vi "test_riccat_01Ni.vi"() -> (3 "All Tests Passed":bool)   [LabVIEW 2019]
uses:
  <vilib>/Analysis/Matrix/Datatypes/RealMatrix.ctl
  <vilib>/Rock Robotics/WPI/ThirdParty/JAS_Junk/TrajLib/Trajectory_Library.lvlib
  <vilib>/Analysis/Matrix/NI_Matrix.lvlib
panel:
  out "N1":T1
  out "R1":T1
  out "Q1":T1
  in  "AREF":T1=[[0.25, 1.0, 0.0, 0.0], [0.0, 0.0, 1.0, 0.0], [0.0, 0.0, 0.0, 1.0], [0.0, 0.0, 0.0, 0.0]]
  out "error out 2":errorcluster
  out "Pos Semi Definite":bool
  out "C":T1
  out "Q_Chk_Passed":bool
  out "Q Check":T1
  out "Stable Bad":bool
  out "Bad":bool
  out "Eigenvalues":cdb[](array[numeric])
  out "error out":errorcluster
  out "Error":bool
  out "Iterations":i32
  out "Elapsed \nTime MS":dbl
  out "ZERO":T1
  out "X  Answer":T1
  in  "R":T1=[[0.25]]
  in  "Q":T1=[[1.0, 0.0, 0.0, 0.0], [0.0, 0.0, 0.0, 0.0], [0.0, 0.0, 0.0, 0.0], [0.0, 0.0, 0.0, 0.0]]
  in  "B":T1=[[0.0], [0.0], [0.0], [1.0]]
  in  "A":T1=[[0.5, 1.0, 0.0, 0.0], [0.0, 0.0, 1.0, 0.0], [0.0, 0.0, 0.0, 1.0], [0.0, 0.0, 0.0, 0.0]]
  # "Test 1: non-invertible A\n  // Example 2 of \"On the Numerical Solution of the Discrete-Time Algebraic\n  // Riccati Equation\""
  # "int n1 = 4, m1 = 1;"
  # "Example = F"
  # "MatrixXd A1(n1, n1), B1(n1, m1), Q1(n1, n1), R1(m1, m1);"
  # "A1 << 0.5, 1, 0, 0, \n          0, 0, 1, 0, \n          0, 0, 0, 1, \n          0, 0, 0, 0;"
  # "B1 << 0, \n        0, \n        0, \n        1;"
  # "Example G1"
  # "Example H"
  # "Solution weight ??"
  # "Q1 << 1, 0, 0, 0, \n        0, 0, 0, 0, \n        0, 0, 0, 0, \n        0, 0, 0, 0;"
  # "Example G2"
  # "Cost ??"
  # "R1 << 0.25;"
  # "0.25, 1, 0, 0, \n0,      0, 1, 0, \n0,      0, 0, 1, \n0,      0, 0, 0;"
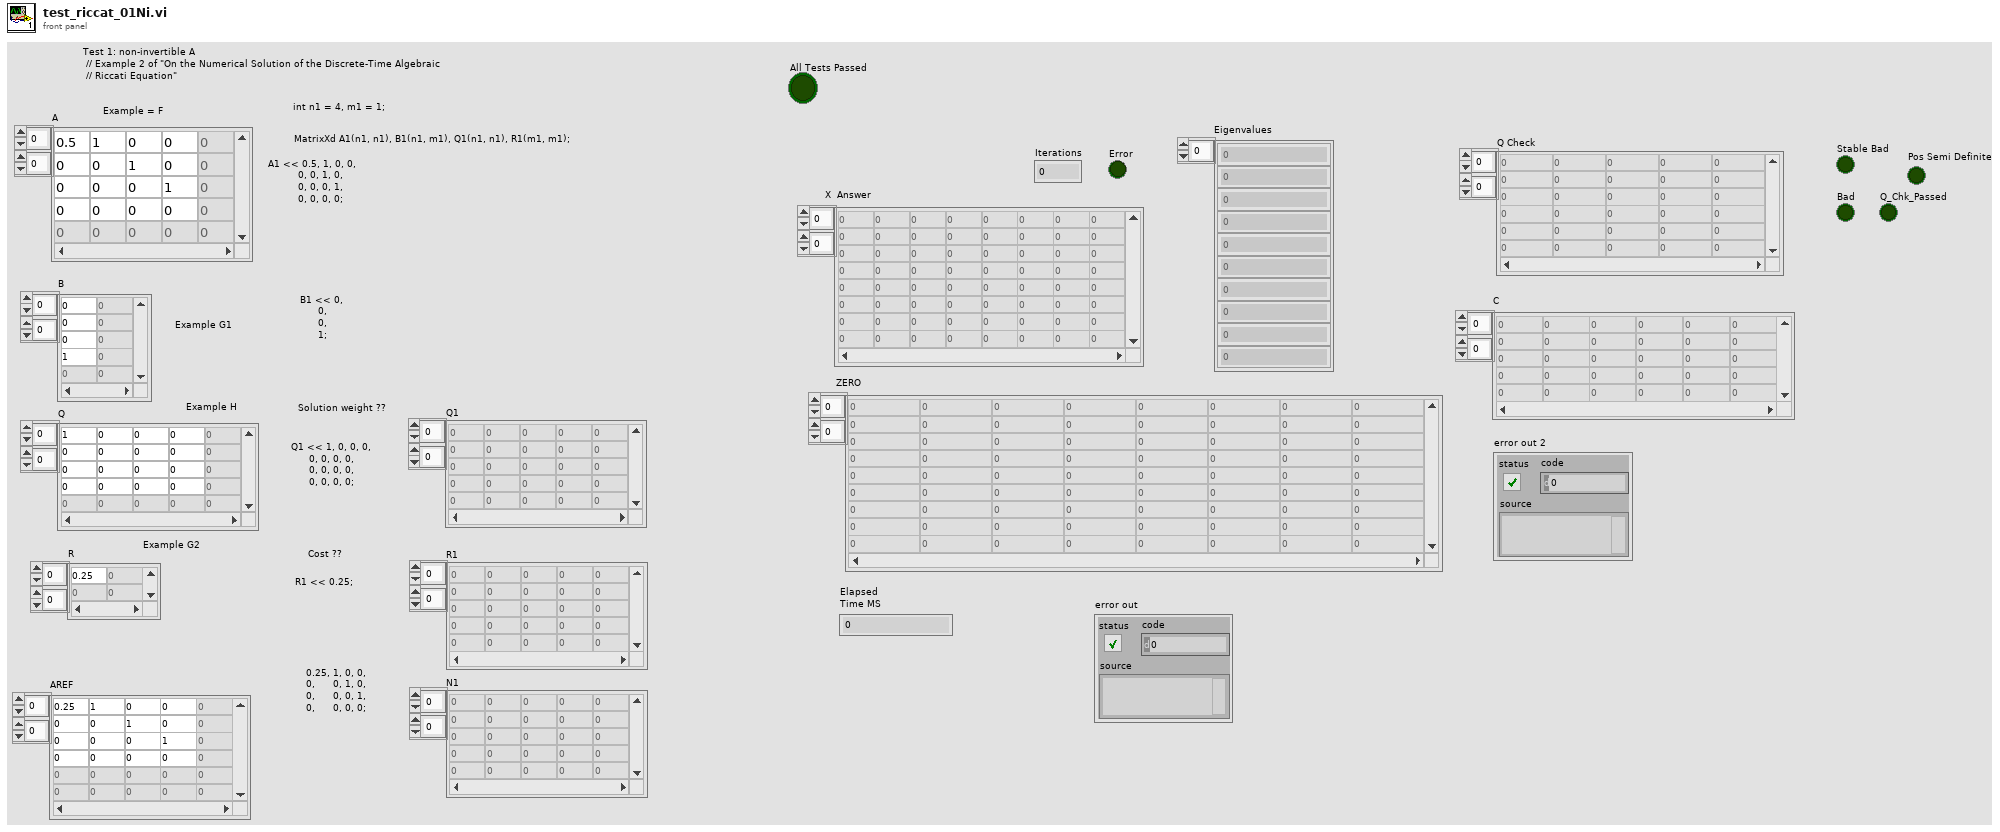
[diagram p1: front panel]
types:
  T1 = typedef "NI_Matrix.lvlib/RealMatrix.ctl" = dbl[][]
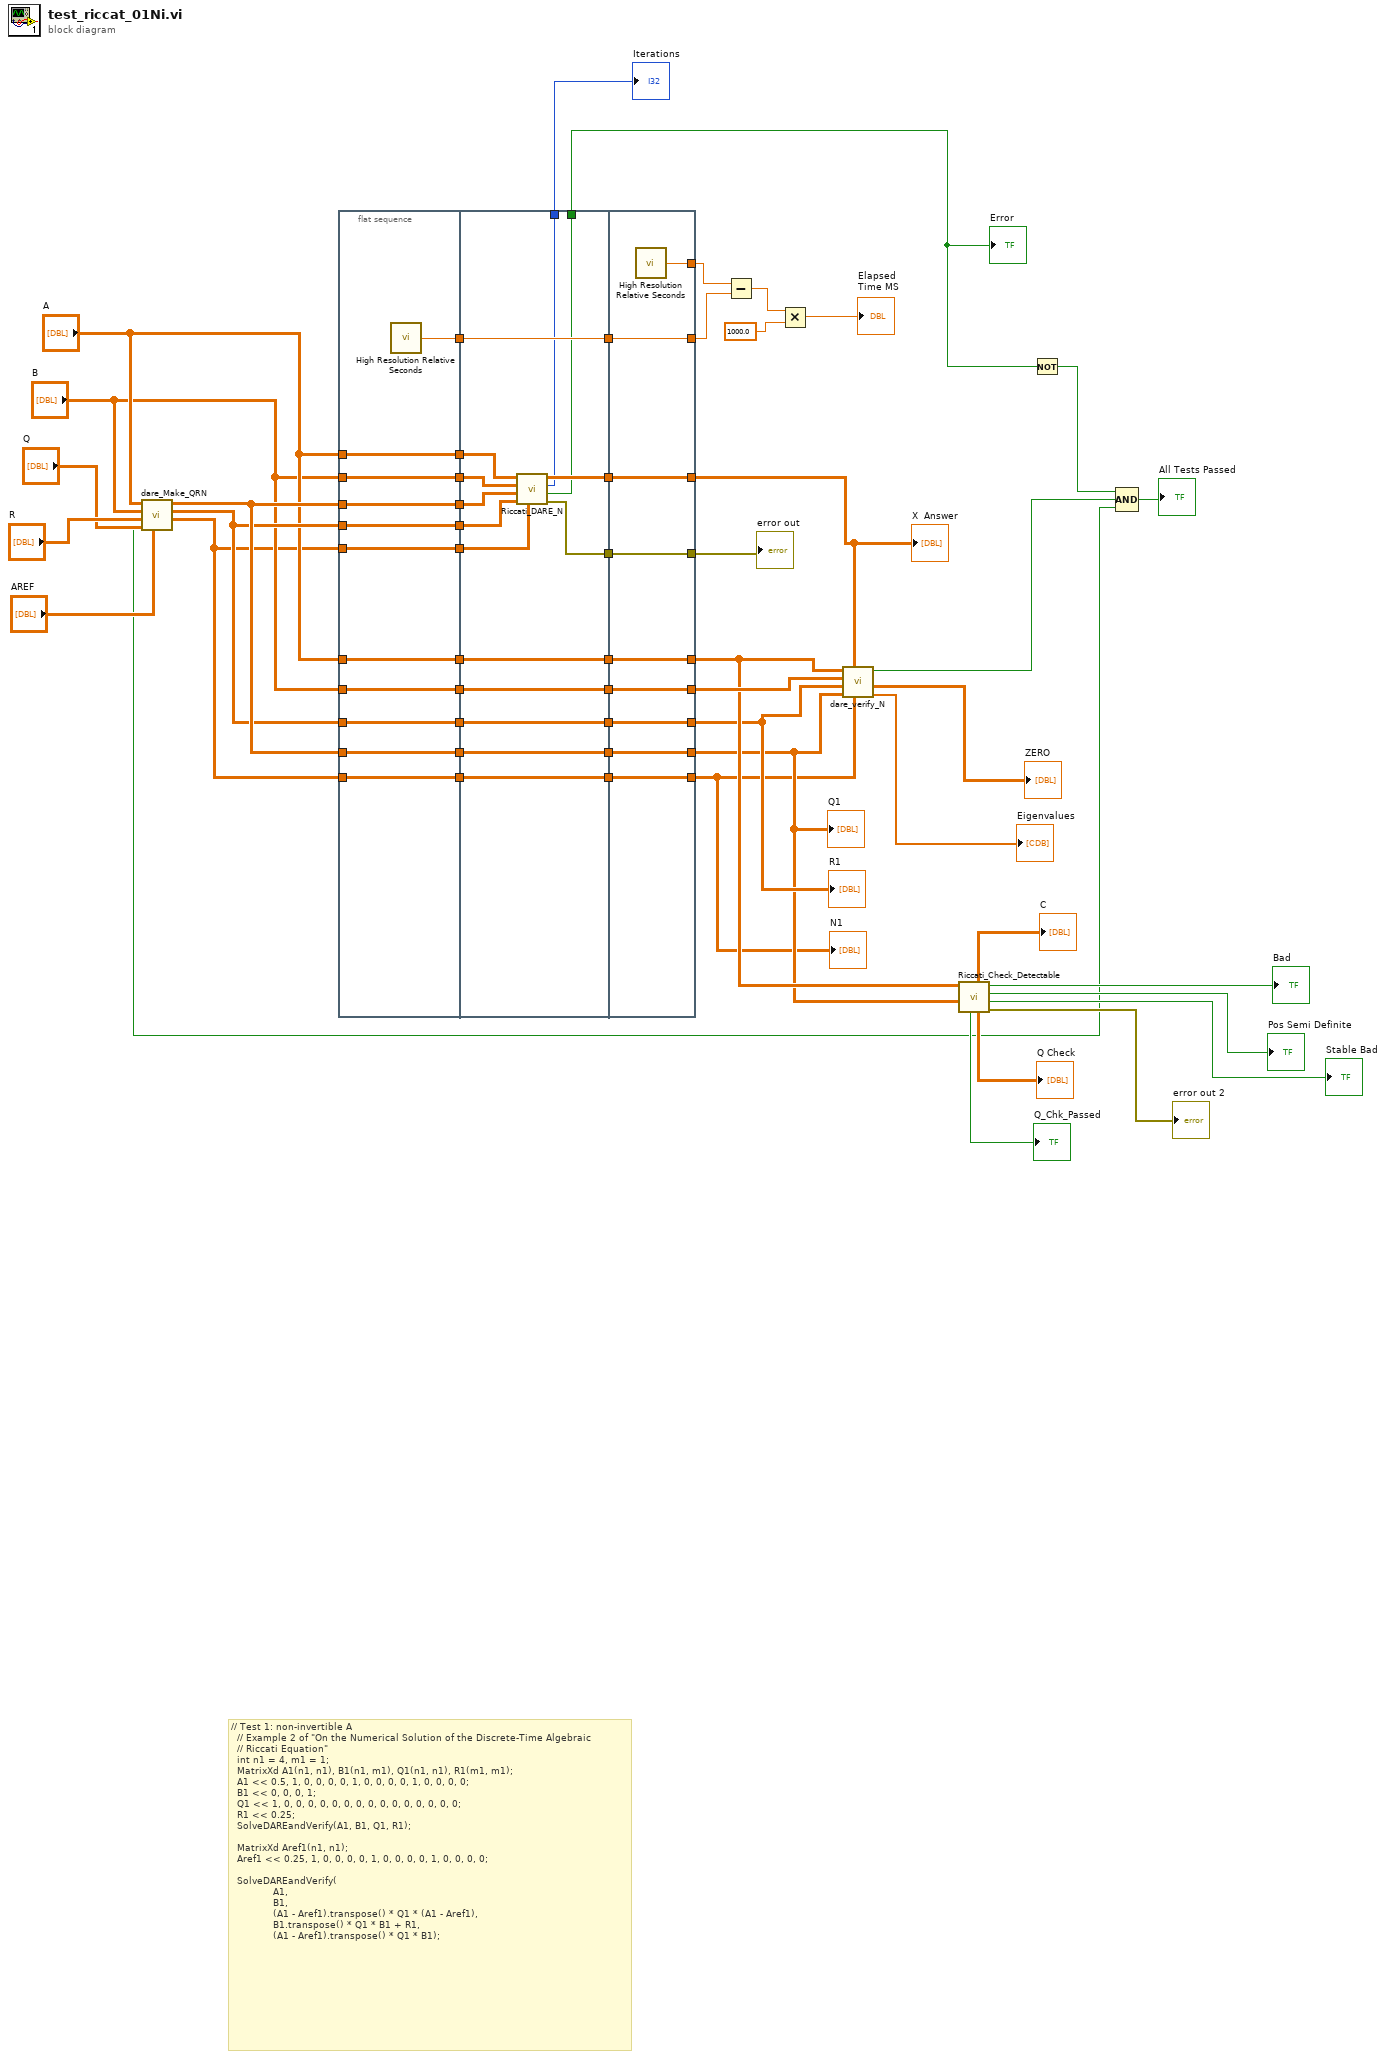
[diagram p0: block diagram]
diagram:
  # "// Test 1: non-invertible A\n  // Example 2 of \"On the Numerical Solution of the Discrete-Time Algebraic\n  // Riccati Equation\"\n  int n1 = 4, m1 = 1;\n  MatrixXd A1(n1, n1), B1(n1, m1), Q1(n1, n1), R1(m1, m1);\n  A1 << 0.5, 1, 0, 0, 0, 0, 1, 0, 0, 0, 0, 1, 0, 0, 0, 0;\n  B1 << 0, 0, 0, 1;\n  Q1 << 1, 0, 0, 0, 0, 0, 0, 0, 0, 0, 0, 0, 0, 0, 0, 0;\n  R1 << 0.25;\n  SolveDAREandVerify(A1, B1, Q1, R1);\n\n  MatrixXd Aref1(n1, n1);\n  Aref1 << 0.25, 1, 0, 0, 0, 0, 1, 0, 0, 0, 0, 1, 0, 0, 0, 0;\n\n  SolveDAREandVerify(\n              A1, \n              B1, \n              (A1 - Aref1).transpose() * Q1 * (A1 - Aref1),\n              B1.transpose() * Q1 * B1 + R1, \n              (A1 - Aref1).transpose() * Q1 * B1);"
  n1 = call "dare_Make_QRN.vi"("AREF"="AREF", "Q"="Q", "R"="R", "B"="B", "A"="A") -> ("Good"=w5:bool, "N1"=w4:T1, "R1"=w12:T1, "Q1"=w13:T1)  [unwired: 3 in]
  n2 = flat-sequence {
    tunnel: "B" -> [w60]
    tunnel: "A" -> [w61]
    tunnel: "B" -> [w62]
    tunnel: w13 -> [w63]
    tunnel: "A" -> [w64]
    tunnel: w12 -> [w65]
    tunnel: [w65] -> w54
    tunnel: [w64] -> w53
    tunnel: [w63] -> w52
    tunnel: [w62] -> w51
    tunnel: [w61] -> w50
    tunnel: [w60] -> w49
    tunnel: w12 -> [w59]
    tunnel: [w59] -> w44
    tunnel: w13 -> [w58]
    tunnel: [w58] -> w43
    tunnel: [w57] -> w38
    tunnel: [w56] -> w11
    tunnel: w4 -> [w56]
    tunnel: w4 -> [w55]
    tunnel: [w55] -> w1
    tunnel: w54 -> [w80]
    tunnel: w53 -> [w78]
    tunnel: w52 -> [w77]
    tunnel: w51 -> [w76]
    tunnel: w50 -> [w75]
    tunnel: w49 -> [w74]
    tunnel: [w79] -> w48
    tunnel: [w75] -> w47
    tunnel: [w74] -> w46
    tunnel: [w73] -> w45
    tunnel: w44 -> [w73]
    tunnel: w43 -> [w72]
    tunnel: [w72] -> w42
    tunnel: [w71] -> w39
    tunnel: w38 -> [w71]
    tunnel: [w70] -> w34
    tunnel: [w69] -> w33
    tunnel: [w68] -> w32
    tunnel: w11 -> [w67]
    tunnel: [w66] -> w2
    tunnel: w1 -> [w66]
    tunnel: [w87] -> w29
    tunnel: [w88] -> w23
    tunnel: [w89] -> w30
    tunnel: w48 -> [w89]
    tunnel: w47 -> [w88]
    tunnel: w46 -> [w87]
    tunnel: [w86] -> w22
    tunnel: w45 -> [w86]
    tunnel: [w85] -> w20
    tunnel: w42 -> [w85]
    tunnel: [w84] -> w41
    tunnel: [w83] -> w40
    tunnel: w39 -> [w83]
    tunnel: w32 -> [w82]
    tunnel: [w82] -> w31
    tunnel: [w81] -> w3
    tunnel: w2 -> [w81]
    frame #0 {
      n3 = call <vilib>:"High Resolution Relative Seconds.vi"() -> ("relative seconds"=w57:dbl)
    }
    frame #1 {
      n4 = call <vilib>:"Riccati_DARE_N.vi"("N"=w67, "R"=w80, "Q"=w77, "B"=w76, "A"=w78) -> ("error out"=w68:errorcluster, "Error"=w69:bool, "Iterations"=w70:i32, "Answer"=w79:T1)  [unwired: 3 in]
    }
    frame #2 {
      n5 = call <vilib>:"High Resolution Relative Seconds.vi"() -> ("relative seconds"=w84:dbl)
    }
  }
  n6 = Subtract(x=w41, y=w40) -> (x-y=w37:dbl)
  n7 = Multiply(x=w37, y=1000.0) -> (x*y=→"Elapsed \nTime MS":dbl)
  n8 = call "dare_verify_N.vi"("N"=w3, "Answer"=w30, "Q"=w20, "R"=w22, "B"=w29, "A"=w23) -> ("Eigenvalues"=→"Eigenvalues":cdb[], "ZERO"=→"ZERO":T1, "Passed"=w25:bool)  [unwired: 3 in]
  n9 = call <vilib>:"Riccati_Check_Detectable.vi"("Q"=w20, "A"=w23) -> ("error out"=→"error out 2":errorcluster, "Stable Bad"=→"Stable Bad":bool, "Pos Semi Definite"=→"Pos Semi Definite":bool, "Bad"=→"Bad":bool, "Q_Check"=→"Q Check":T1, "C"=→"C":T1, "Q_Chk_Passed"=→"Q_Chk_Passed":bool)  [unwired: 3 in]
  n10 = Not(x=w33) -> (.not. x?=w26:bool)
  n11 = Compound Arithmetic op=AND(w26, w25, w5) -> (→"All Tests Passed":bool)
  "X  Answer" <- w30
  "Iterations" <- w34
  "Error" <- w33
  "error out" <- w31
  "Q1" <- w20
  "R1" <- w22
  "N1" <- w3
